vi "Find Strings Common Root.vi"(8 "Error In":errorcluster, 9 "Suffix Break Character (_)":string="_", 11 "String Array":string[](array[string])) -> (0 "Error Out":errorcluster, 1 "Folder Suffixes":string[](array[string]), 3 "Common Root":string)   [LabVIEW 2021, in "Strings.lvlib"]
uses:
  Strings.lvlib
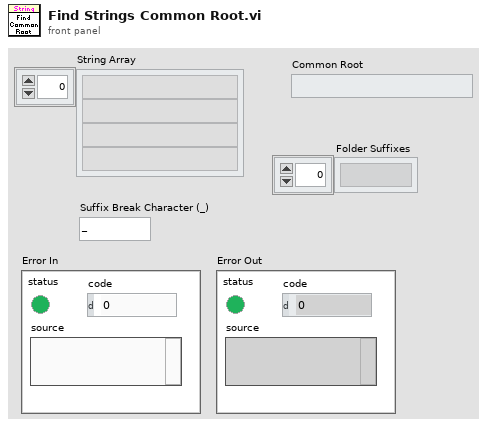
[diagram p1: front panel]
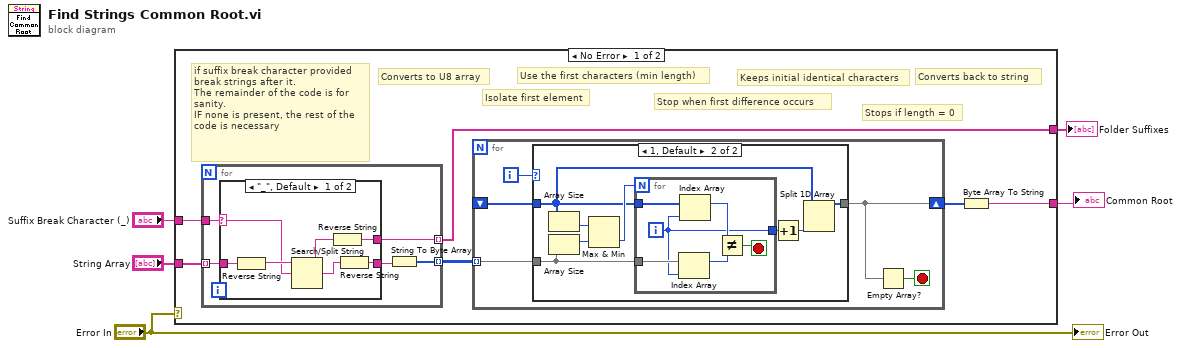
[diagram p0: block diagram]
diagram:
  n1 = case shown="No Error" "Error In" {
    tunnel: "String Array" -> [w11 _]
    tunnel: [w8 _] -> w3
    tunnel: "Suffix Break Character (_)" -> [w7 _]
    tunnel: [w6 _] -> w1
    frame No Error {
      # "if suffix break character provided\nbreak strings after it.\nThe remainder of the code is for sanity.\nIF none is present, the rest of the code is necessary"
      # "Converts back to string"
      # "Stops if length = 0"
      # "Keeps initial identical characters"
      # "Stop when first difference occurs"
      # "Use the first characters (min length)"
      # "Isolate first element"
      # "Converts to U8 array"
      n2 = for {
        tunnel: w11 -> [w14] mode=indexing
        tunnel: [w16] -> w10 mode=indexing
        tunnel: w7 -> [w15]
        tunnel: [w12] -> w6 mode=indexing
        n3 = case shown="\"_\", Default" w15 {
          selector: w15 -> [w21 _]
          tunnel: w14 -> [w23 w24]
          tunnel: [w19 w24] -> w13
          tunnel: [w17 _] -> w12
          frame "_", Default {
            n4 = Reverse String(1:w23) -> (0:w22:string)
            n5 = Search/Split String(string=w22, search string/char (-)=w21) -> (substring before match=w18:string, match + rest of string=w20:string)  [unwired: 1 in, 1 out]
            n6 = Reverse String(1:w18) -> (0:w17:string)
            n7 = Reverse String(1:w20) -> (0:w19:string)
          }
          frame "" {
          }
        }
        n8 = String To Byte Array(string=w13) -> (unsigned byte array=w16:u8[])
      }
      n9 = for {
        tunnel: w10 -> [w28] mode=indexing
        shift-right: [w26] -> w9
        shift-left: _ -> [w27]
        i -> [w29]
        stop <- w25 stop-if-true
        n10 = case shown="1, Default" w29 {
          tunnel: w28 -> [w30 w35]
          tunnel: [w30 w32] -> w26
          tunnel: w27 -> [_ w34]
          frame 0 {
          }
          frame 1, Default {
            n11 = Array Size(array=w34) -> (size(s)=w38:i32)
            n12 = Array Size(array=w35) -> (size(s)=w37:i32)
            n13 = Max & Min(x=w38, y=w37) -> (min(x,y)=w36:i32)  [unwired: 1 out]
            n14 = for {
              N: w36 -> [_]
              tunnel: w34 -> [w44]
              tunnel: w35 -> [w43]
              tunnel: [w39] -> w33
              i -> [w39]
              stop <- w40 stop-if-true
              n15 = Index Array(array=w43, index=w39) -> (element=w41:u8)
              n16 = Index Array(array=w44, index=w39) -> (element=w42:u8)
              n17 = Not Equal?(x=w42, y=w41) -> (x != y?=w40:bool)
            }
            n18 = Increment(x=w33) -> (x+1=w31:i32)
            n19 = Split 1D Array(array=w34, index=w31) -> (first subarray=w32:u8[])  [unwired: 1 out]
          }
        }
        n20 = Empty Array?(array=w26) -> (empty?=w25:bool)
      }
      n21 = Byte Array To String(unsigned byte array=w9) -> (string=w8:string)
    }
    frame Error {
    }
  }
  "Common Root" <- w3
  "Folder Suffixes" <- w1
  "Error Out" <- "Error In"
